vi "ConvertSCPIValueToBoolean.vi"(11 "SCPI Value":string) -> (3 "Boolean":bool)   [LabVIEW 2009, in "Keithley-6482-Visa.lvlib"]
uses:
  <instrlib>/Keithley-6482-Visa9.0/Keithley-6482-Visa.lvlib
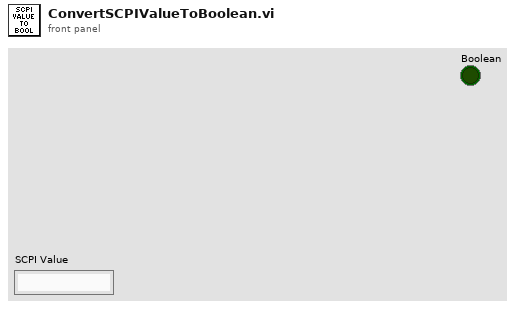
[diagram p1: front panel]
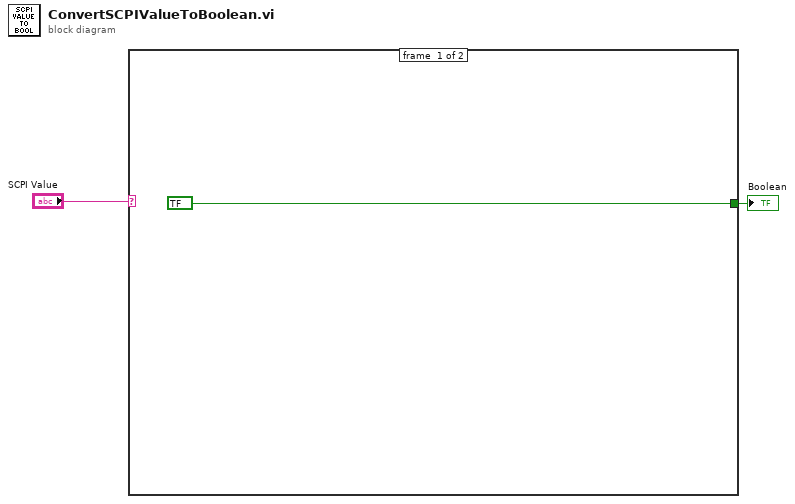
[diagram p0: block diagram]
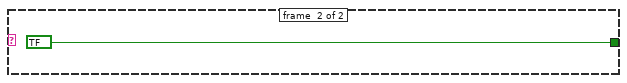
[diagram p2: hidden frame]
diagram:
  n1 = case shown="\"ON\"" "SCPI Value" {
    tunnel: [bool ? bool ?] -> w1
    frame #0 {
    }
    frame #1 {
    }
  }
  "Boolean" <- w1
